vi "get first and last value.vi"(10 "Array":dbl[](array[numeric])) -> (2 "Freq info":T1 {"resolution" format="%#_6p"; "Delta" format="%#_6p"; "Min" format="%#_6p"; "Max" format="%#_6p"})   [LabVIEW 2020]
uses:
  analyse freq.ctl
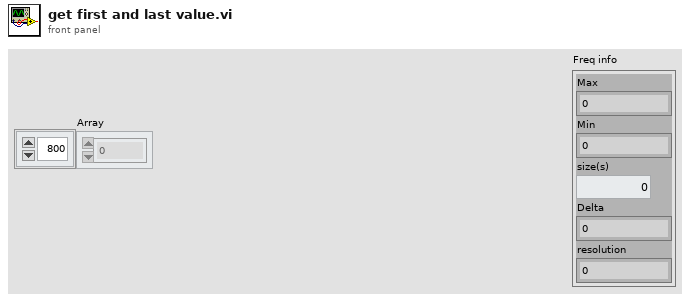
[diagram p1: front panel]
types:
  T1 = typedef "analyse freq.ctl" = cluster{"Max":dbl, "Min":dbl, "size(s)":i32, "Delta":dbl, "resolution":dbl}
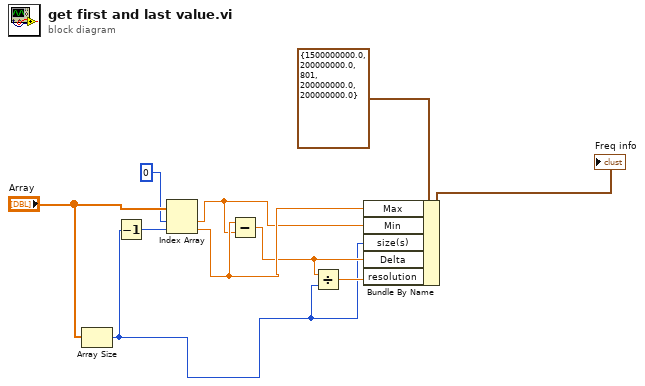
[diagram p0: block diagram]
diagram:
  n1 = Array Size(array="Array") -> (size(s)=w1:i32)
  n2 = Decrement(x=w1) -> (x-1=w9:i32)
  n3 = Index Array(array="Array", index #1=0 ("index"), index #2=w9) -> (element #1=w4:dbl, element #2=w5:dbl)
  n4 = Subtract(x=w5, y=w4) -> (x-y=w3:dbl)
  n5 = Divide(x=w3, y=w1) -> (x/y=w2:dbl)
  n6 = Bundle By Name(cluster=T1 {"Max"=1500000000.0, "Min"=200000000.0, "size(s)"=801, "Delta"=200000000.0, "resolution"=200000000.0} ("Freq info"), "Max"=w5, "Min"=w4, "size(s)"=w1, "Delta"=w3, "resolution"=w2) -> (→"Freq info":T1)
